vi "Report Errors.vi"(8 "error in":errorcluster, 9 "Iterator Error":errorcluster, 10 "Caller Enqueuer in":refnum<class "Message Enqueuer.lvclass">, 11 "Iterator Actor in":refnum<class "Iterator Actor.lvclass">) -> (0 "error out":errorcluster, 3 "Iterator Actor out":refnum<class "Iterator Actor.lvclass">)   [LabVIEW 2016, in "Iterator Actor.lvlib" / "Iterator Actor.lvclass"]
uses:
  Iterator Actor.lvclass
  <vilib>/ActorFramework/Message Enqueuer/Message Enqueuer.lvclass
  Iterator Actor.lvclass/Iterator Actor.ctl
  Iterator Actor Abstract Messages/Iterator Report Error Msg/Iterator Report Error Msg.lvclass
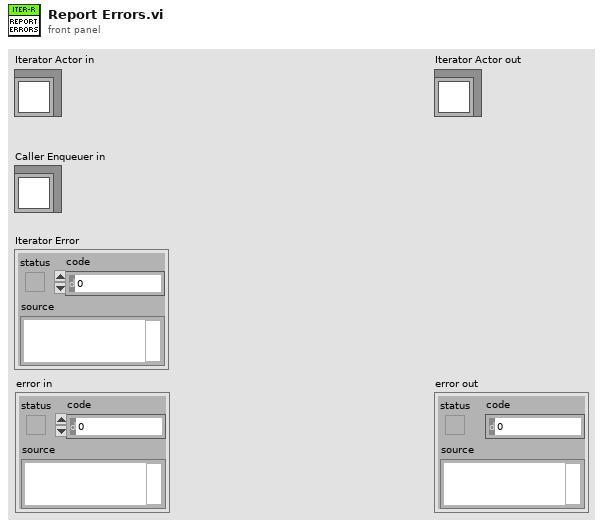
[diagram p1: front panel]
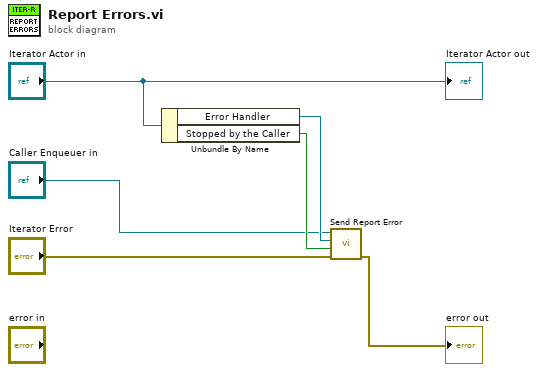
[diagram p0: block diagram]
diagram:
  n1 = Unbundle By Name("Iterator Actor in") -> ("Error Handler"=w4:refnum<class "Iterator Report Error Msg.lvclass">, "Stopped by the Caller"=w5:bool)
  n2 = call "Send Report Error.vi"("error in (no error)"="Iterator Error", "Stopped by the Caller?"=w5, "Caller Error Handler"=w4, "Caller Enqueuer in"="Caller Enqueuer in") -> ("error out"=→"error out":errorcluster)  [unwired: 6 in, 1 out]
  "Iterator Actor out" <- "Iterator Actor in"
